vi "Close Log File.vi"(8 "error in (no error)":errorcluster, 11 "Log File in":refnum<class "Log File.lvclass">) -> (0 "error out":errorcluster, 3 "File Path":path)   [LabVIEW 2015, in "Waveform Data Logger Engine.lvlib" / "Log File.lvclass"]
uses:
  Log File.lvclass
  Log File.lvclass/Log File.ctl
  TDMS Log File/TDMS Log File.lvclass
  TDMS Log File/TDMS Log File.lvclass/TDMS Log File.ctl
  Text Log File/Text Log File.lvclass
  Text Log File/Text Log File.lvclass/Text Log File.ctl
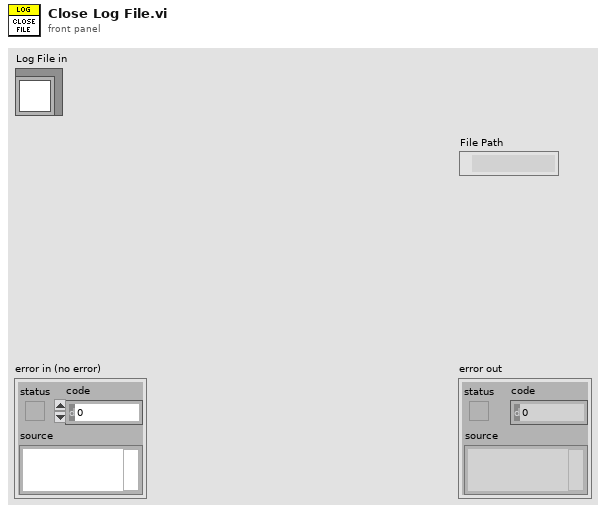
[diagram p1: front panel]
types:
  T1 = typedef "Waveform Data Logger Engine.lvlib/Log File.lvclass/Log File Type.ctl" = enum16{"Default", "TDMS", "Text"}
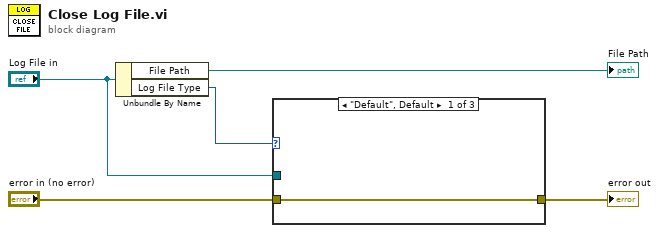
[diagram p0: block diagram]
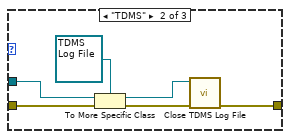
[diagram p2: hidden frame]
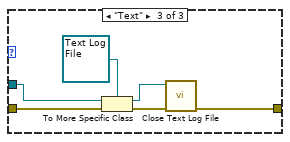
[diagram p3: hidden frame]
diagram:
  n1 = Unbundle By Name("Log File in") -> ("File Path"=→"File Path":path, "Log File Type"=w4:T1)
  n2 = case shown="\"Default\", Default" w4 {
    tunnel: "error in (no error)" -> [w6 w12 w17]
    tunnel: [w6 w7 w18] -> w2
    tunnel: "Log File in" -> [_ w11 w15]
    frame "Default", Default {
    }
    frame "TDMS" {
      n3 = To More Specific Class(target class=refnum<class "TDMS Log File.lvclass"> refnum ("TDMS Log File.lvclass"), reference=w11, error in=w12) -> (specific class reference=w9:refnum<class "TDMS Log File.lvclass">, error out=w8:errorcluster)
      n4 = call "Close TDMS Log File.vi"("error in (no error)"=w8, "TDMS Log File in"=w9) -> ("error out"=w7:errorcluster)  [unwired: 8 in, 1 out]
    }
    frame "Text" {
      n5 = To More Specific Class(target class=refnum<class "Text Log File.lvclass"> refnum ("Text Log File.lvclass"), reference=w15, error in=w17) -> (specific class reference=w13:refnum<class "Text Log File.lvclass">, error out=w16:errorcluster)
      n6 = call "Close Text Log File.vi"("error in (no error)"=w16, "Text Log File in"=w13) -> ("error out"=w18:errorcluster)  [unwired: 8 in, 1 out]
    }
  }
  "error out" <- w2
